vi "myRIO_BRig_RT_dataBlock_iBlock__R.vi"() -> (2 "output_iBlock__R":i32)   [LabVIEW 2014]
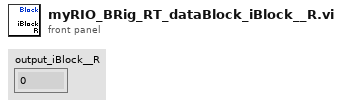
[diagram p1: front panel]
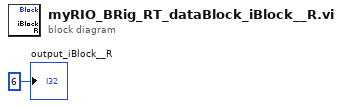
[diagram p0: block diagram]
diagram:
  "output_iBlock__R" <- 6 ("output_iBlock")
